vi "Discover Power Supply GPIB.vi"(11 "ADDRESS IN":string) -> (2 "PSn Model":string)   [LabVIEW 2018]
uses:
  Station References Global.vi
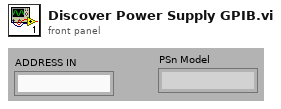
[diagram p1: front panel]
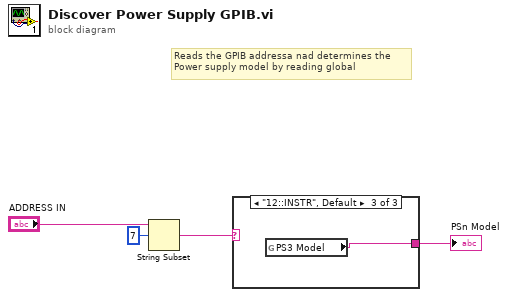
[diagram p0: block diagram]
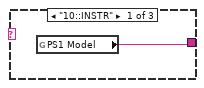
[diagram p2: hidden frame]
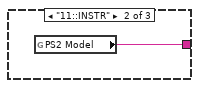
[diagram p3: hidden frame]
diagram:
  # "Reads the GPIB addressa nad determines the \nPower supply model by reading global"
  n1 = String Subset(string="ADDRESS IN", offset (0)=7) -> (substring=w3:string)  [unwired: 1 in]
  n2 = case shown="\"12::INSTR\", Default" w3 {
    tunnel: [w5 w6 w7] -> w2
    frame "10::INSTR" {
      n3 = global read "Station References Global.vi" "PS1 Model"() -> (w5:string)
    }
    frame "11::INSTR" {
      n4 = global read "Station References Global.vi" "PS2 Model"() -> (w6:string)
    }
    frame "12::INSTR", Default {
      n5 = global read "Station References Global.vi" "PS3 Model"() -> (w7:string)
    }
  }
  "PSn Model" <- w2
